vi "Shift Cursor.vi"(6 "chip select (1st chip)":enum16{"1st chip", "2nd chip"}(ring), 8 "error in (no error)":errorcluster, 10 "direction":enum16{"left", "right"}(ring), 11 "LCD in":u32) -> (0 "error out":errorcluster, 3 "LCD out":u32)   [LabVIEW 2015, in "HD44780 FPGA.lvlib"]
doc: "Shifts the cursor position to the left or right."
uses:
  <vilib>/EmbeddedDisplay/Hitachi HD44780/FPGA/HD44780 FPGA.lvlib
  <vilib>/EmbeddedDisplay/Hitachi HD44780/Common/HD44780 Common.lvlib
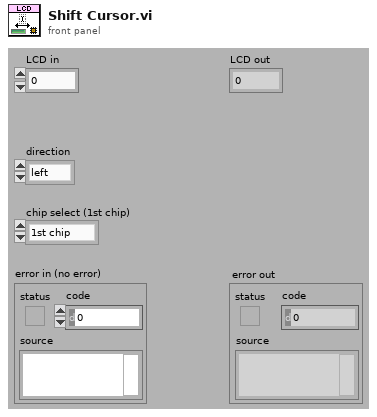
[diagram p1: front panel]
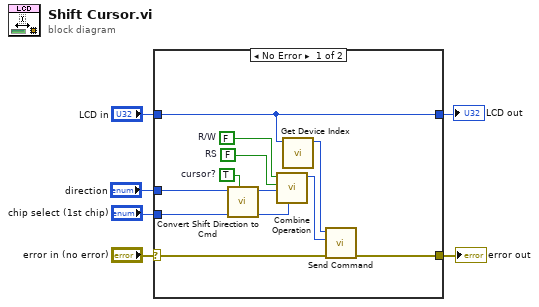
[diagram p0: block diagram]
diagram:
  n1 = case shown="No Error" "error in (no error)" {
    selector: "error in (no error)" -> [w12 w19]
    tunnel: [w11 w19] -> w5
    tunnel: "LCD in" -> [w7 w18]
    tunnel: "direction" -> [w10 _]
    tunnel: "chip select (1st chip)" -> [w9 _]
    tunnel: [w7 w18] -> w1
    frame No Error {
      w14 = FALSE  # R/W
      w17 = TRUE  # cursor?
      w15 = FALSE  # RS
      n2 = call <vilib>:"Convert Shift Direction to Cmd.vi"("cursor?"=w17, "direction"=w10) -> ("LCD data/cmd"=w16:u8)  [unwired: 9 in]
      n3 = call <vilib>:"Combine Operation.vi"("chip select  (1st chip)"=w9, "cmd/data (0)"=w16, "RS"=w15, "R/W"=w14) -> ("output"=w13:u32)  [unwired: 7 in]
      n4 = call <vilib>:"Get Device Index.vi"("LCD in"=w7) -> ("device index"=w8:i8)  [unwired: 10 in]
      n5 = call <vilib>:"Send Command.vi"("error in (no error)"=w12, "operation"=w13, "device index"=w8) -> ("error out"=w11:errorcluster)  [unwired: 6 in, 2 out]
    }
    frame Error {
    }
  }
  "error out" <- w5
  "LCD out" <- w1
